vi "MUSIQC_trap_control_trap1.vi"() -> ()   [LabVIEW 2009]
uses:
  <vilib>/DAQmx/configure/timing.llb/DAQmx Timing (Sample Clock).vi
  <vilib>/DAQmx/create/channels.llb/DAQmx Create Channel (CI-Count Edges).vi
  <vilib>/DAQmx/read.llb/DAQmx Read (Counter U32 1Chan 1Samp).vi
  <vilib>/Utility/file.llb/Write To Spreadsheet File (I64).vi
  Program Files/National Instruments/LabVIEW 2009/resource/objmgr/daqmx.rc
  <vilib>/Analysis/NI_AALBase.lvlib
panel:
  out "Ion":bool
  out "Counts":u32
  in  "Oven":bool
  in  "Orange":bool
  in  "Sample rate":dbl=50.0 format="%0.2f"
  in  "snap":bool
  in  "Threshold":u32
  in  "Auto Load":bool
  in  "RF":bool
  in  "Blue":bool
  in  "Red":bool
  out "Mean/Variance":dbl
  out "Variance":dbl format="%0.2f"
  out "Mean":dbl format="%0.2f"
  in  "Samples per averaging\nblock":i32=100 min=1 step=1
  in  "stop":bool
  out "PMT Counts":cluster{"mean":dbl, u32}(graph)
  out "Counts total":dbl
  # "Trap 1"
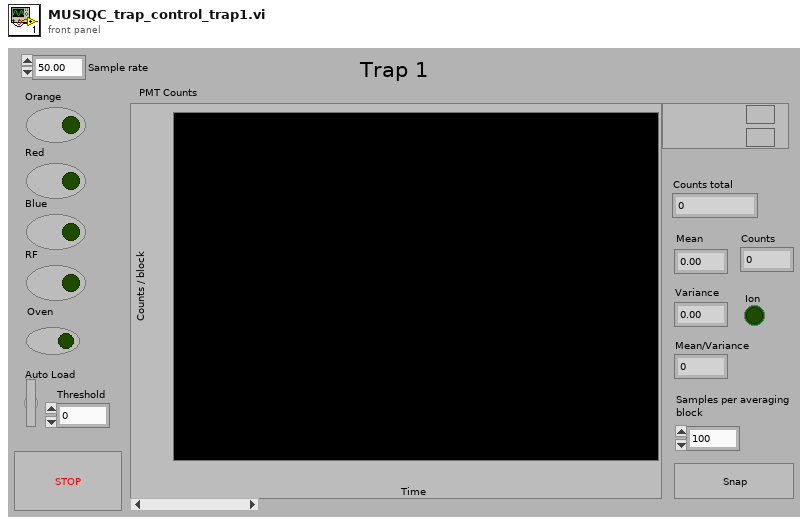
[diagram p1: front panel]
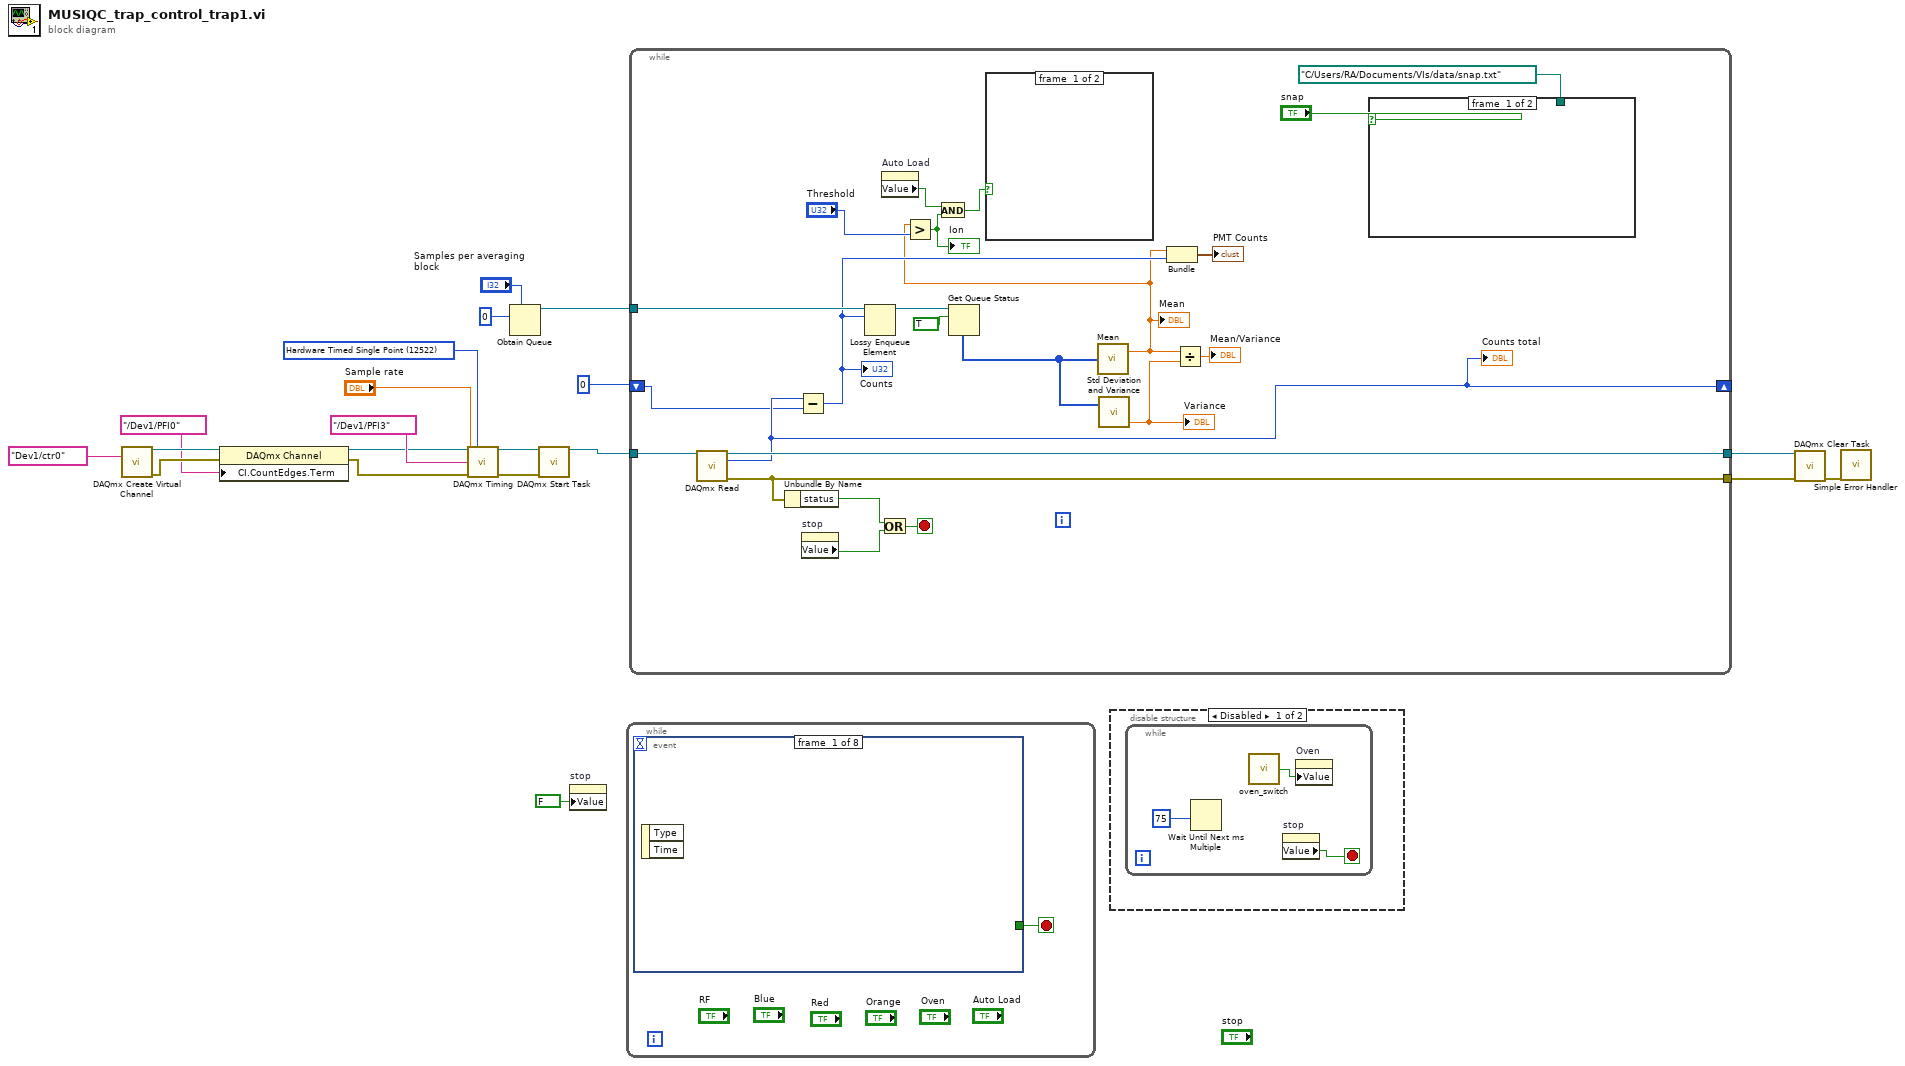
[diagram p0: block diagram]
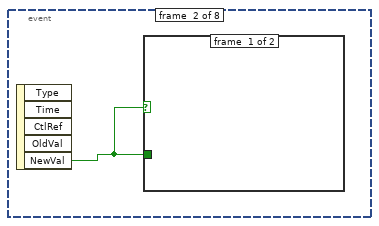
[diagram p3: hidden frame]
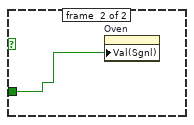
[diagram p4: hidden frame]
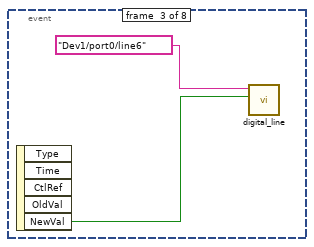
[diagram p5: hidden frame]
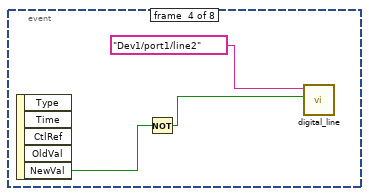
[diagram p6: hidden frame]
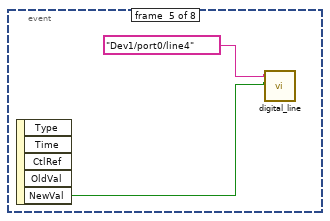
[diagram p7: hidden frame]
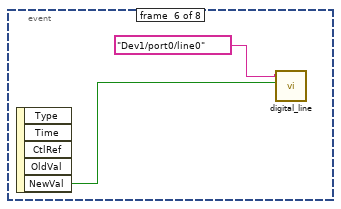
[diagram p8: hidden frame]
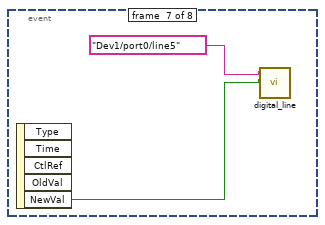
[diagram p9: hidden frame]
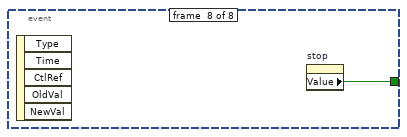
[diagram p10: hidden frame]
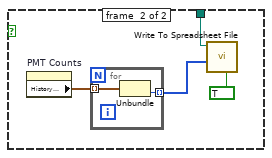
[diagram p11: hidden frame]
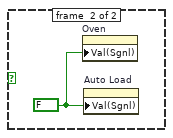
[diagram p12: hidden frame]
diagram:
  w1 = 12522 items=["Finite Samples"=10178, "Continuous Samples"=10123, "Hardware Timed Single Point"=12522] ("sample mode")
  n1 = call-poly <vilib>:"DAQmx Create Virtual Channel.vi"("counter"=tag "Dev1/ctr0") -> ("task out"=w10:refnum<k21>, "error out"=w9:errorcluster)  [unwired: 13 in]
  n2 = property class="DAQmx Channel"(reference=w10, error in=w9, "CI.CountEdges.Term"=tag "/Dev1/PFI0") -> (reference out=w12:refnum<k21>, error out=w11:errorcluster)
  n3 = call-poly <vilib>:"DAQmx Timing.vi"("task/channels in"=w12, "sample mode"=w1, "rate"="Sample rate", "source"=tag "/Dev1/PFI3", "error in"=w11) -> ("task out"=w19:refnum<k21>, "error out"=w18:errorcluster)  [unwired: 9 in]
  n4 = Obtain Queue(max queue size (-1, unlimited)="Samples per averaging\nblock", element data type=u32 0) -> (queue out=w5:refnum<queue>)  [unwired: 3 in, 2 out]
  n5 = call <vilib>:"DAQmx Start Task.vi"("task/channels in"=w19, "error in"=w18) -> ("task out"=w13:refnum<k21>)  [unwired: 12 in, 1 out]
  n6 = property on="stop" class="Bool (strict)"("Value"=FALSE ("stop")) -> ()  [unwired: 2 in, 2 out]
  n7 = while {
    stop <- w21 stop-if-true
    n8 = event shown="[1] \"Auto Load\": Value Change" {
      selector: _ -> [_ _ _ _ _ _ _ _]
      dyn-events: _ -> [_ _ _ _ _ _ _ _]
      timeout: _ -> [_ _ _ _ _ _ _ _]
      tunnel: [_ _ _ _ _ _ _ w35] -> w21
      event #0 {
        n9 = event-data() -> ()  [unwired: 1 in, 2 out]
      }
      event #1 {
        n10 = event-data() -> ("NewVal"=w22:bool)  [unwired: 1 in, 4 out]
        n11 = case shown="True" w22 {
          tunnel: w22 -> [_ w23]
          frame #0 {
          }
          frame #1 {
            n12 = property on="Oven" class="Bool (strict)"("Val(Sgnl)"=w23) -> ()  [unwired: 2 in, 2 out]
          }
        }
      }
      event #2 {
        n13 = event-data() -> ("NewVal"=w24:bool)  [unwired: 1 in, 4 out]
        n14 = call "digital_line.vi"("NewVal"=w24, "lines"=tag "Dev1/port0/line6") -> ()  [unwired: 2 in]
      }
      event #3 {
        n15 = event-data() -> ("NewVal"=w26:bool)  [unwired: 1 in, 4 out]
        n16 = Not(x=w26) -> (.not. x?=w27:bool)
        n17 = call "digital_line.vi"("NewVal"=w27, "lines"=tag "Dev1/port1/line2") -> ()  [unwired: 2 in]
      }
      event #4 {
        n18 = event-data() -> ("NewVal"=w29:bool)  [unwired: 1 in, 4 out]
        n19 = call "digital_line.vi"("NewVal"=w29, "lines"=tag "Dev1/port0/line4") -> ()  [unwired: 2 in]
      }
      event #5 {
        n20 = event-data() -> ("NewVal"=w31:bool)  [unwired: 1 in, 4 out]
        n21 = call "digital_line.vi"("NewVal"=w31, "lines"=tag "Dev1/port0/line0") -> ()  [unwired: 2 in]
      }
      event #6 {
        n22 = event-data() -> ("NewVal"=w33:bool)  [unwired: 1 in, 4 out]
        n23 = call "digital_line.vi"("NewVal"=w33, "lines"=tag "Dev1/port0/line5") -> ()  [unwired: 2 in]
      }
      event #7 {
        n24 = event-data() -> ()  [unwired: 1 in, 5 out]
        n25 = property on="stop" class="Bool (strict)"() -> ("Value"=w35:bool)  [unwired: 2 in, 2 out]
      }
    }
  }
  n26 = while {
    shift-right: [w40] -> _
    shift-left: u32 0 -> [w39]
    tunnel: [w56] -> w15
    tunnel: [w55] -> w14
    tunnel: w13 -> [w54]
    tunnel: w5 -> [w53]
    stop <- w58 stop-if-true
    n27 = call-poly <vilib>:"DAQmx Read.vi"("task/channels in"=w54) -> ("task out"=w55:refnum<k21>, "data"=w40:u32, "error out"=w56:errorcluster)  [unwired: 12 in]
    "Counts total" <- w40
    n28 = Unbundle By Name(w56) -> ("status"=w57:bool)
    n29 = Subtract(x=w40, y=w39) -> (x-y=w38:u32)
    "Counts" <- w38
    n30 = property on="stop" class="Bool (strict)"() -> ("Value"=w48:bool)  [unwired: 2 in, 2 out]
    n31 = Lossy Enqueue Element(queue=w53, element=w38) -> (queue out=w52:refnum<queue>)  [unwired: 1 in, 3 out]
    n32 = Or(x=w57, y=w48) -> (x .or. y?=w58:bool)
    n33 = property on="Auto Load" class="Bool (strict)"() -> ("Value"=w45:bool)  [unwired: 2 in, 2 out]
    n34 = Get Queue Status(queue=w52, return elements? (F)=TRUE) -> (elements=w42:u32[])  [unwired: 1 in, 7 out]
    n35 = call <vilib>:"Mean.vi"("X"=w42) -> ("mean"=w36:dbl)  [unwired: 1 out]
    "Mean" <- w36
    n36 = Greater?(x=w36, y="Threshold") -> (0:w46:bool)
    "Ion" <- w46
    n37 = And(x=w45, y=w46) -> (x .and. y?=w44:bool)
    n38 = case shown="True" w44 {
      frame #0 {
      }
      frame #1 {
        w65 = FALSE ("Auto Load")
        n39 = property on="Oven" class="Bool (strict)"("Val(Sgnl)"=w65) -> ()  [unwired: 2 in, 2 out]
        n40 = property on="Auto Load" class="Bool (strict)"("Val(Sgnl)"=w65) -> ()  [unwired: 2 in, 2 out]
      }
    }
    n41 = call <vilib>:"Std Deviation and Variance.vi"("X"=w42) -> ("variance"=w50:dbl)  [unwired: 1 in, 2 out]
    "Variance" <- w50
    n42 = Bundle("mean"=w36, w38) -> (→"PMT Counts":cluster{"mean":dbl, u32})  [unwired: 1 in]
    n43 = Divide(x=w36, y=w50) -> (x/y=→"Mean/Variance":dbl)
    n44 = case shown="True" "snap" {
      tunnel: path "C:/Users/RA/Documents/VIs/data/snap.txt" ("file path (dialog if empty)") -> [_ w61]
      frame #0 {
      }
      frame #1 {
        n45 = property on="PMT Counts" class="WFChart (strict)"() -> ("History Data"=w60:cluster{"mean":dbl, u32}[])  [unwired: 2 in, 2 out]
        n46 = for {
          tunnel: w60 -> [w64] mode=indexing
          tunnel: [w63] -> w59 mode=indexing
          n47 = Unbundle(w64) -> (w63:u32)  [unwired: 1 out]
        }
        n48 = call-poly <vilib>:"Write To Spreadsheet File.vi"("transpose? (no:F)"=TRUE, "1D data"=w59, "file path (dialog if empty)"=w61) -> ()  [unwired: 5 in, 1 out]
      }
    }
  }
  n49 = disable-structure shown="Disabled" {
    frame #0 {
      n50 = while {
        stop <- w66 stop-if-true
        n51 = Wait Until Next ms Multiple(millisecond multiple=u32 75) -> ()  [unwired: 1 out]
        n52 = call "oven_switch.vi"() -> ("Final state"=w68:bool)  [unwired: 2 in]
        n53 = property on="stop" class="Bool (strict)"() -> ("Value"=w66:bool)  [unwired: 2 in, 2 out]
        n54 = property on="Oven" class="Bool (strict)"("Value"=w68) -> ()  [unwired: 2 in, 2 out]
      }
    }
    frame #1 {
    }
  }
  n55 = call <vilib>:"DAQmx Clear Task.vi"("task in"=w14, "error in"=w15) -> ("error out"=w3:errorcluster)  [unwired: 13 in]
  n56 = call <vilib>:"Simple Error Handler.vi"("error in (no error)"=w3) -> ()  [unwired: 4 in, 5 out]
